vi "Configure Systems Copy.vi"() -> ()   [LabVIEW 2009, in "POLARIS BME DG.lvlib" / "BME_DG_System.lvclass"]
uses:
  DG Classes/BME_DG_System/BME_DG_System.lvclass
  DetectDG.ctl
  System DG Selection.ctl
  LV-BME Interface/BME_DG_TriggerSettings.ctl
  LV-BME Interface/ClockSource.ctl
  SG08_Settings.ctl
  LV-BME Interface/BME_DG_V2TriggerSettings.ctl
  MSBus.ctl
  LV-BME Interface/ChnlSettings.ctl
  Go_Done_Chnl_Settings.ctl
  SG08_Chnl_Settings.ctl
  Chnl Settings Complete.ctl
  Card Config.ctl
  <vilib>/Utility/xml.llb/Write to XML File(array).vi
  <vilib>/Utility/error.llb/DialogType.ctl
  POLARIS BME DG.lvlib
panel:
  in  "stop":bool
  in  "Tab Control":T1(tab)=enum."Define Channels"
  in  "InstalledDGs":T2[](array[typedef])
  in  "Select System":u16(ring) items=["MiraSync", "POLARISTrigger"]
  in  "Systems":T3[](array[typedef])
  in  "Selected DG":u16(ring) items=["0", "1", "2"]
  in  "Add":bool
  in  "Remove":bool
  in  "Empty Systems":bool
  in  "DetectDGs":bool
  in  "Find Card by Name":u16(ring) items=["MiraSync", "FE PP", "A1 Hapt", "A1 Neben", "A2 Haupt", "A2 Neben", "A2 PP", "A2 PP, A2.5", "A3 Haupt", "A4 Haupt"]
  in  "Card Config":T9(array[cluster]) {"Advanced Settings"."Trigger on MS Bus" format="%04x" items=["Local Primary0x1"=1, "Local Secondary0x2"=2, "Local Force 0x4"=4, "Resynchronize 0x8"=8, "Master Prim. 0x10"=16, "Master Sec. 0x20"=32, "Master Force  0x40"=64, "System Clock 0x80"=128, "Delay Clock 0x100"=256, "Inhibit Local 0x200"=512, "Start Local 0x400"=1024, "Start Bus 0x800"=2048, "Step Back Local 0x1000"=4096, "Step Back Bus 0x2000"=8192, "RunCircle 0x4000"=16384, "SyncReload 0x8000"=32768, "From E 0x10000"=65536, "From F 0x20000"=131072, "From Bus 0x40000"=262144]; "Advanced Settings"."Force Trigger (µs)" min=0.0 format="%.6f"; "SG08_Settings"."StepBackTime (µs)" min=0.0 format="%.6f"; "SG08_Settings"."Gate Delay (µs)" format="%.3f"; "SG08_Settings"."Gate Level" min=-2.5 max=2.5 format="%.3g"; "Base Settings"."Gate Divider" min=1 max=1000000; "Base Settings"."Clock Source" items=["Internal Oscillator"=1, "External Trigger"=2, "Trigger-> Oscillator"=3, "MasterSlave Bus"=4]; "Base Settings"."Inhibit(µs)" format="%#_11g"}
  in  "Find Card by Chnl":u16(ring) items=["MiraSyncT", "MiraSyncA", "MiraSyncB", "Delay Offset", "Pulspicker On", "Pulspicker Off", "10 Hz Target", "A1 PC On", "A1 PC Off", "Fast PC On", "Dazzler", "Kompressor", "A2 LDD", "A2 PC On", "A2 PC Off", "Oszi", "Kamera", "A5", "A2 PP1 On", "A2 PP1 Off", "A2 PP2 On", "A2 PP2 Off", "A2.5 LDD", "Keppis A3", "A3 LDD", "A3 PC On", "A3 PC Off", "A4 LDD", "A3-Kamera", "A4-Kamera", "Oszi", "A2 PP1 On", "A2 PP2 Off", "A3 LDD", "A4 LDD"]
  in  "Find Chnl":u16(ring) items=["MiraSyncT", "MiraSyncA", "MiraSyncB", "Delay Offset", "Pulspicker On", "Pulspicker Off", "10 Hz Target", "A1 PC On", "A1 PC Off", "Fast PC On", "Dazzler", "Kompressor", "A2 LDD", "A2 PC On", "A2 PC Off", "Oszi", "Kamera", "A5", "A2 PP1 On", "A2 PP1 Off", "A2 PP2 On", "A2 PP2 Off", "A2.5 LDD", "Keppis A3", "A3 LDD", "A3 PC On", "A3 PC Off", "A4 LDD", "A3-Kamera", "A4-Kamera", "Oszi", "A2 PP1 On", "A2 PP2 Off", "A3 LDD", "A4 LDD"]
  in  "Copy Chnl Names":bool=TRUE
  in  "Chnls":T13(array[cluster]) {"ChnParameter"."Delay (µs)" min=0.0 max=100000000.0 format="%.5f"; "G08_Chnl_Settings"."Pulse Width (µs)" min=0.0 max=8947840.0 format="%#.6f"; "Go and Done Signal"."Done Signal" format="%04x" items=["Local Primary"=1, "Local Secondary"=2, "Local Force"=4, "Master Primary"=16]; "Go and Done Signal"."Go Signal" format="%04x" items=["Local Primary0x1"=1, "Local Secondary0x2"=2, "Local Force 0x4"=4, "Resynchronize 0x8"=8, "Master Prim. 0x10"=16, "Master Sec. 0x20"=32, "Master Force  0x40"=64, "System Clock 0x80"=128, "Delay Clock 0x100"=256, "Inhibit Local 0x200"=512, "Start Local 0x400"=1024, "Start Bus 0x800"=2048, "Step Back Local 0x1000"=4096, "Step Back Bus 0x2000"=8192, "RunCircle 0x4000"=16384, "SyncReload 0x8000"=32768, "From E 0x10000"=65536, "From F 0x20000"=131072, "From Bus 0x40000"=262144]}
  out "Last Change":timestamp=timestamp(3422440183.453125 s since 1904-01-01)
  in  "Save":bool
  in  "Load":bool=TRUE
  in  "Config File":path
  # "DGNr"
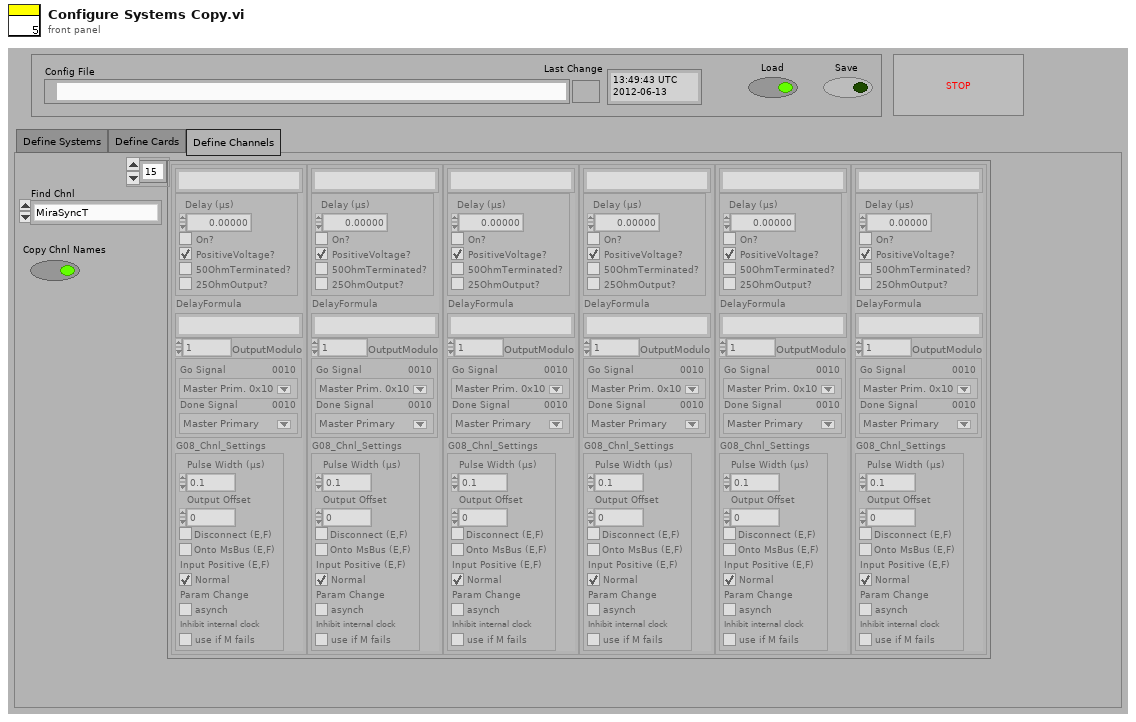
[diagram p1: front panel]
types:
  T1 = enum32{"Define Systems", "Define Cards", "Define Channels"}
  T2 = typedef "POLARIS BME DG.lvlib/DetectDG.ctl" = cluster{"DG_Number":i32, "DG_Product":i32, "Product Name":string, "Bus_Number":i32, "Slot_Number":i32, "Master":bool}
  T3 = typedef "POLARIS BME DG.lvlib/System DG Selection.ctl" = cluster{"Selected System DGs":T2[], "Name":string}
  T4 = typedef "POLARIS BME DG.lvlib/BME_DG_TriggerSettings.ctl" = cluster{"Clock Source":T5, " clock modulo":u32, "TriggerEnabled?":bool, "trigger modulo ":i32, "InputTerminated?":bool, "Inhibit(µs)":dbl, "TriggerLevel":dbl, "PresetValue":i32, "InternalTrigger?":bool, "InternalArm?":bool, "SWTrigger?":bool, "RisingEdge?":bool, "StopOnPreset?":bool, "ResetWhenDone?":bool, "Gate Divider":i32, "PositiveGate?":bool}
  T5 = typedef "POLARIS BME DG.lvlib/ClockSource.ctl" = i32
  T6 = typedef "POLARIS BME DG.lvlib/SG08_Settings.ctl" = cluster{"Gate Terminate":bool, "Gate Level":dbl, "Gate Delay (µs)":dbl, "StepBackTime (µs)":dbl, "Burst Counter":u32, "Trigger Divider":u32, "Trigger Multiplier":u32}
  T7 = typedef "POLARIS BME DG.lvlib/BME_DG_V2TriggerSettings.ctl" = cluster{"Trigger on MS Bus":T8, "Force Trigger (µs)":dbl, "Gate Type":bool, "Synchronize Gate":bool}
  T8 = typedef "POLARIS BME DG.lvlib/MSBus.ctl" = u32
  T9 = cluster{"Logical Name":string, "Base Settings":T4, "SG08_Settings":T6, "Channel Names":string[], "Advanced Settings":T7}[]
  T10 = typedef "POLARIS BME DG.lvlib/ChnlSettings.ctl" = cluster{" Delay (µs)":dbl, "On?":bool, "PositiveVoltage?":bool, "50OhmTerminated? ":bool, "25OhmOutput?":bool}
  T11 = typedef "POLARIS BME DG.lvlib/Go_Done_Chnl_Settings.ctl" = cluster{"Go Signal":T8, "Done Signal":u32}
  T12 = typedef "POLARIS BME DG.lvlib/SG08_Chnl_Settings.ctl" = cluster{"Pulse Width (µs)":dbl, "Output Offset":u32, "Disconnect (E,F)":bool, "Onto MsBus (E,F)":bool, "Input Positive (E,F)":bool, "Param Change":bool, "Inhibit internal clock":bool}
  T13 = cluster{"Channel Name":string, "ChnParameter":T10, "DelayFormula":string, "OutputModulo":i32, "Go and Done Signal":T11, "G08_Chnl_Settings":T12}[]
  T14 = typedef "POLARIS BME DG.lvlib/Chnl Settings Complete.ctl" = cluster{"Channel Name":string, "ChnParameter":T10, "DelayFormula":string, "OutputModulo":i32, "Go and Done Signal":T11, "G08_Chnl_Settings":T12}
  T15 = typedef "POLARIS BME DG.lvlib/Card Config.ctl" = cluster{"Logical Name":string, "Base Settings":T4, "SG08_Settings":T6, "Channel Names":string[], "Advanced Settings":T7}
  T16 = typedef "DialogType.ctl" = u16
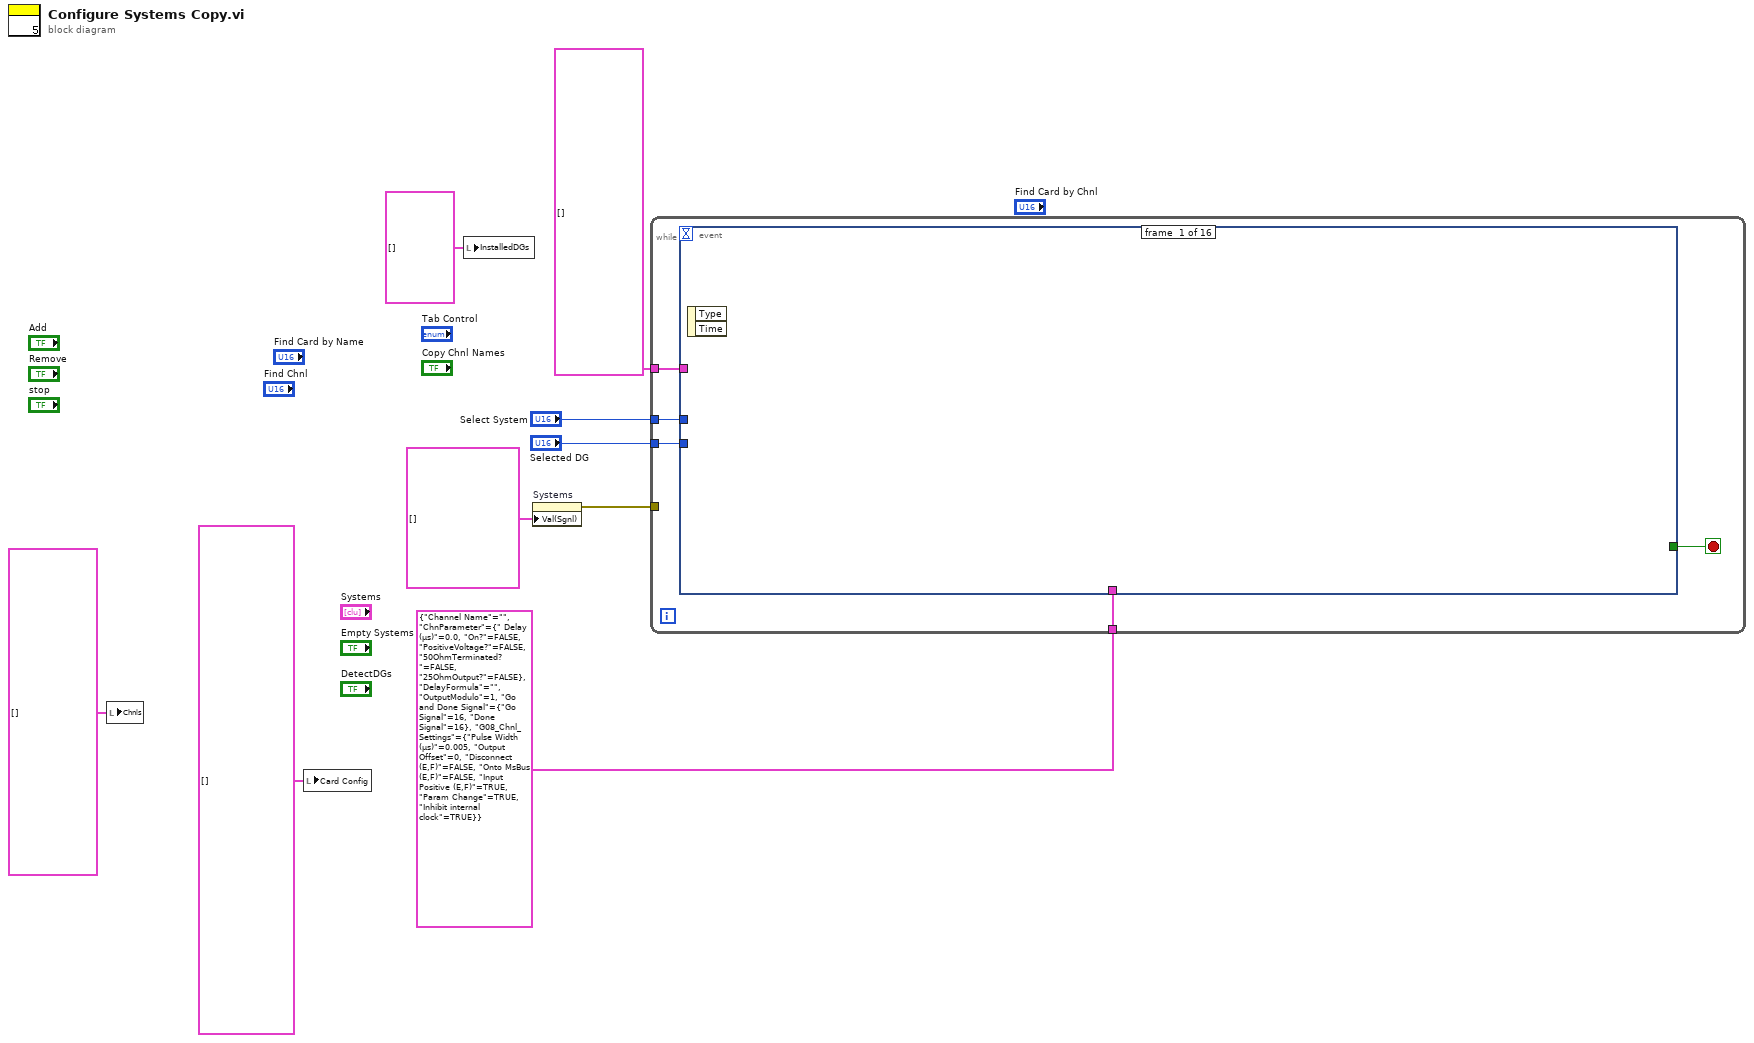
[diagram p0: block diagram]
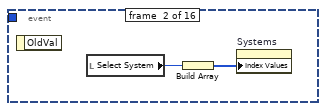
[diagram p2: hidden frame]
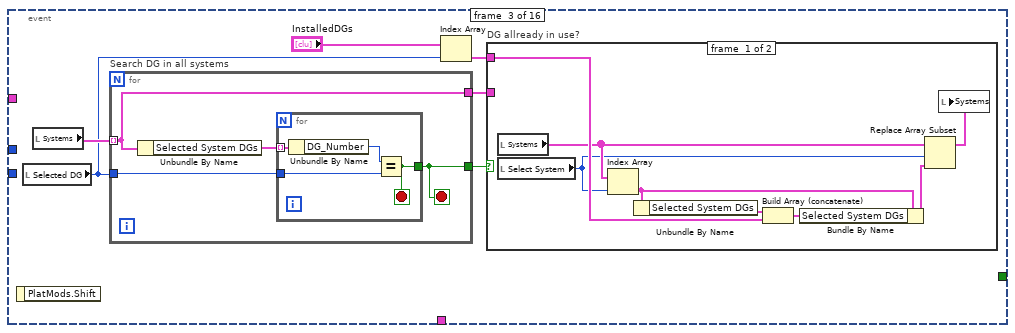
[diagram p3: hidden frame]
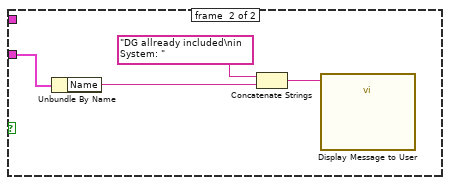
[diagram p4: hidden frame]
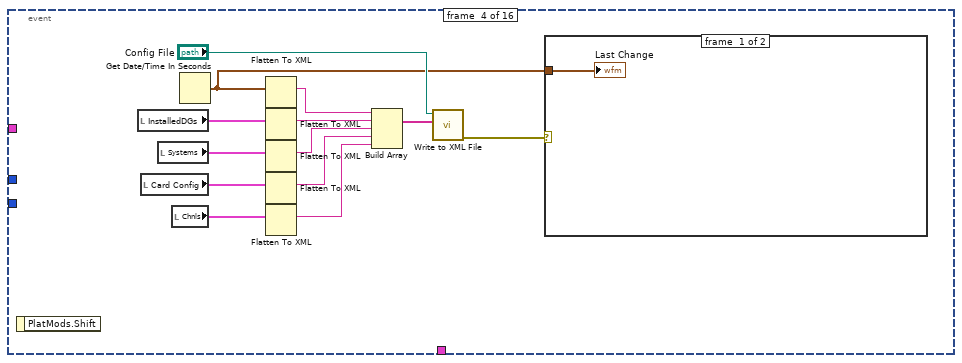
[diagram p5: hidden frame]
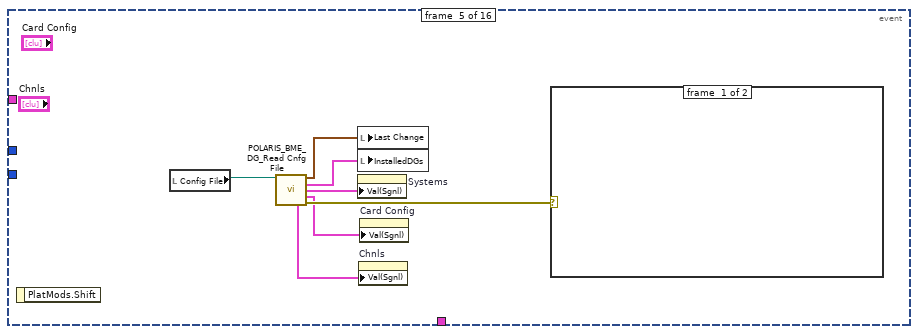
[diagram p7: hidden frame]
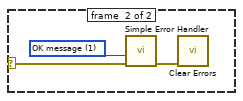
[diagram p8: hidden frame]
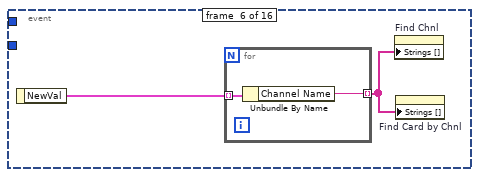
[diagram p9: hidden frame]
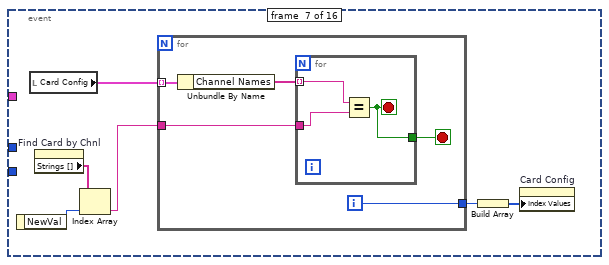
[diagram p10: hidden frame]
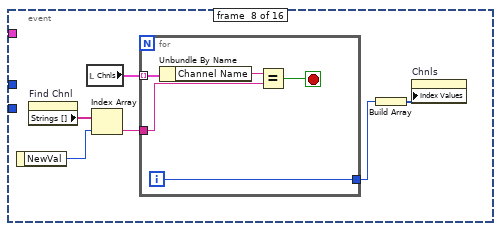
[diagram p11: hidden frame]
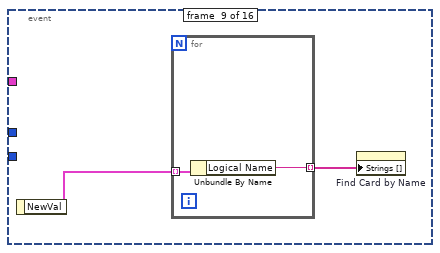
[diagram p12: hidden frame]
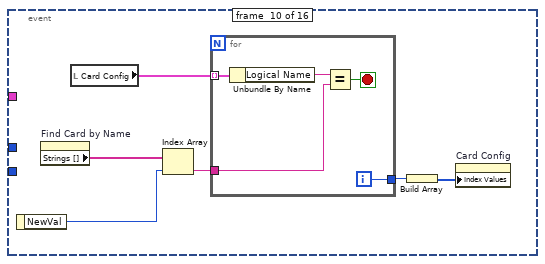
[diagram p13: hidden frame]
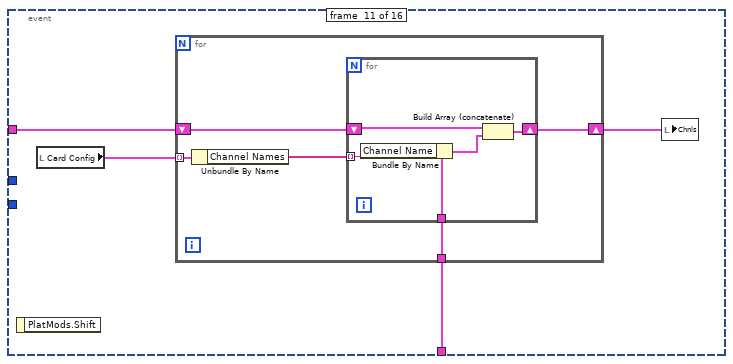
[diagram p14: hidden frame]
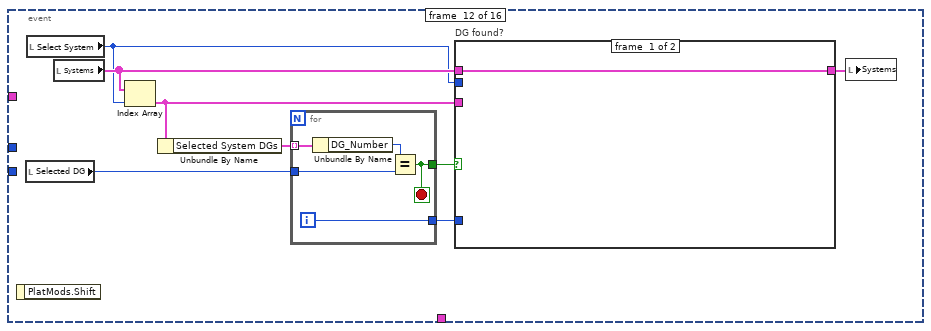
[diagram p15: hidden frame]
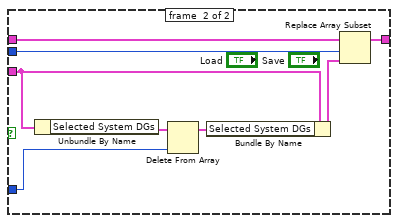
[diagram p16: hidden frame]
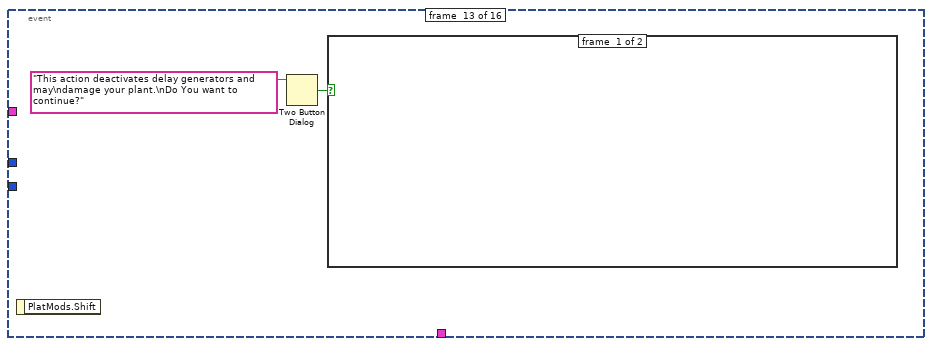
[diagram p17: hidden frame]
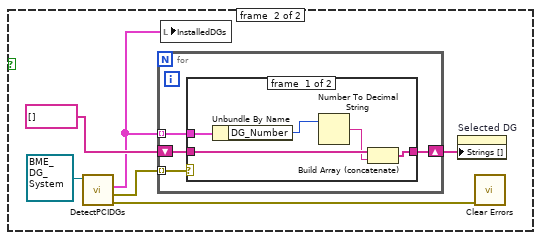
[diagram p18: hidden frame]
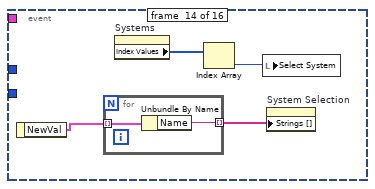
[diagram p20: hidden frame]
diagram:
  n1 = local write "Chnls"(T14[] [] ("Chnls")) -> ()
  n2 = local write "Card Config"(T15[] [] ("Card Config")) -> ()
  n3 = local write "InstalledDGs"(T2[] [] ("InstalledDGs")) -> ()
  n4 = property on="Systems" class="Arr (strict)"("Val(Sgnl)"=T3[] [] ("Value (Signaling)")) -> (error out=w6:errorcluster)  [unwired: 2 in, 1 out]
  n5 = while {
    tunnel: "Select System" -> [w13]
    tunnel: "Selected DG" -> [w12]
    tunnel: w6 -> [_]
    tunnel: T14 {"Channel Name"="", "ChnParameter"={" Delay (µs)"=0.0, "On?"=FALSE, "PositiveVoltage?"=FALSE, "50OhmTerminated? "=FALSE, "25OhmOutput?"=FALSE}, "DelayFormula"="", "OutputModulo"=1, "Go and Done Signal"={"Go Signal"=16, "Done Signal"=16}, "G08_Chnl_Settings"={"Pulse Width (µs)"=0.005, "Output Offset"=0, "Disconnect (E,F)"=FALSE, "Onto MsBus (E,F)"=FALSE, "Input Positive (E,F)"=TRUE, "Param Change"=TRUE, "Inhibit internal clock"=TRUE}} ("Cluster") -> [w11]
    tunnel: T14[] [] -> [w10]
    stop <- w14 stop-if-true
    n6 = event shown="[12] \"DetectDGs\": Mouse Down;  \"DetectDGs\": Key Down" {
      selector: _ -> [_ _ _ _ _ _ _ _ _ _ _ _ _ _ _ _]
      dyn-events: _ -> [_ _ _ _ _ _ _ _ _ _ _ _ _ _ _ _]
      timeout: _ -> [_ _ _ _ _ _ _ _ _ _ _ _ _ _ _ _]
      tunnel: [_ _ _ _ _ _ _ _ _ _ _ _ _ _ _ TRUE] -> w14
      tunnel: w13 -> [_ _ _ _ _ _ _ _ _ _ _ _ _ _ _ _]
      tunnel: w12 -> [_ _ _ _ _ _ _ _ _ _ _ _ _ _ _ _]
      tunnel: w11 -> [_ _ _ _ _ _ _ _ _ _ w112 _ _ _ _ _]
      tunnel: w10 -> [_ _ _ _ _ _ _ _ _ _ w111 _ _ _ _ _]
      event #0 {
        n7 = event-data() -> ()  [unwired: 1 in, 2 out]
      }
      event #1 {
        n8 = event-data() -> ()  [unwired: 1 in, 1 out]
        n9 = local read "Select System"() -> (w16:u16)
        n10 = Build Array(w16) -> (w15:u16[])
        n11 = property on="Systems" class="Arr (strict)"("Index Values"=w15) -> ()  [unwired: 2 in, 2 out]
      }
      event #2 {
        n12 = event-data() -> ()  [unwired: 1 in, 1 out]
        n13 = local read "Selected DG"() -> (w19:u16)
        n14 = local read "Systems"() -> (w22:T3[])
        n15 = for "Search DG in all systems" {
          tunnel: w22 -> [w35] mode=indexing
          tunnel: w19 -> [w37]
          tunnel: [w35] -> w20
          tunnel: [w36] -> w21
          stop <- w36 stop-if-true
          n16 = Unbundle By Name(w35) -> ("Selected System DGs"=w38:T2[])
          n17 = for {
            tunnel: w38 -> [w42] mode=indexing
            tunnel: w37 -> [w41]
            tunnel: [w39] -> w36
            stop <- w39 stop-if-true
            n18 = Unbundle By Name(w42) -> ("DG_Number"=w40:i32)
            n19 = Equal?(x=w40, y=w41) -> (x = y?=w39:bool)
          }
        }
        n20 = Index Array(array="InstalledDGs", index=w19) -> (element=w18:T2)
        n21 = case "DG allready in use?" shown="False" w21 {
          tunnel: w20 -> [_ w34]
          tunnel: w18 -> [w28 _]
          frame #0 {
            n22 = local read "Systems"() -> (w25:T3[])
            n23 = local read "Select System"() -> (w24:u16)
            n24 = Index Array(array=w25, index=w24) -> (element=w23:T3)
            n25 = Unbundle By Name(w23) -> ("Selected System DGs"=w30:T2[])
            n26 = Build Array (concatenate)(w30, w28) -> (w29:T2[])
            n27 = Bundle By Name(cluster=w23, "Selected System DGs"=w29) -> (w26:T3)
            n28 = Replace Array Subset(array=w25, new element=w26, index=w24) -> (w27:T3[])
            n29 = local write "Systems"(w27) -> ()
          }
          frame #1 {
            n30 = Unbundle By Name(w34) -> ("Name"=w31:string)
            n31 = Concatenate Strings("DG allready included\nin System: " ("string"), w31) -> (w33:string)
            n32 = call "Display Message to User"("Message"=w33) -> ()  [unwired: 9 in, 2 out]
          }
        }
      }
      event #3 {
        n33 = event-data() -> ()  [unwired: 1 in, 1 out]
        n34 = local read "InstalledDGs"() -> (w55:T2[])
        n35 = local read "Card Config"() -> (w46:T9)
        n36 = local read "Systems"() -> (w54:T3[])
        n37 = local read "Chnls"() -> (w44:T13)
        n38 = Get Date/Time In Seconds() -> (seconds since 1Jan1904=w48:timestamp)
        n39 = Flatten To XML(anything=w48) -> (xml string=w53:string)
        n40 = Flatten To XML(anything=w55) -> (xml string=w52:string)
        n41 = Flatten To XML(anything=w54) -> (xml string=w51:string)
        n42 = Flatten To XML(anything=w46) -> (xml string=w45:string)
        n43 = Flatten To XML(anything=w44) -> (xml string=w43:string)
        n44 = Build Array(w53, w52, w51, w45, w43) -> (w50:string[])
        n45 = call-poly <vilib>:"Write to XML File.vi"("XML Input"=w50, "XML File Path"="Config File") -> ("error out"=w47:errorcluster)  [unwired: 7 in, 2 out]
        n46 = case shown="No Error" w47 {
          tunnel: w48 -> [w56 _]
          frame #0 {
            "Last Change" <- w56
          }
          frame #1 {
          }
        }
      }
      event #4 {
        n47 = event-data() -> ()  [unwired: 1 in, 1 out]
        n48 = local read "Config File"() -> (w63:path)
        n49 = call "POLARIS_BME_DG_Read Cnfg File.vi"("Config File"=w63) -> ("Last Change"=w62:timestamp, "InstalledDGs"=w61:T2[], "DGSystems"=w60:T3[], "Cards"=w58:T15[], "Chnls"=w57:T14[], "error out"=w59:errorcluster)  [unwired: 9 in]
        n50 = local write "Last Change"(w62) -> ()
        n51 = local write "InstalledDGs"(w61) -> ()
        n52 = property on="Systems" class="Arr (strict)"("Val(Sgnl)"=w60) -> ()  [unwired: 2 in, 2 out]
        n53 = property on="Chnls" class="Arr (strict)"("Val(Sgnl)"=w57) -> ()  [unwired: 2 in, 2 out]
        n54 = property on="Card Config" class="Arr (strict)"("Val(Sgnl)"=w58) -> ()  [unwired: 2 in, 2 out]
        n55 = case shown="Error" w59 {
          selector: w59 -> [_ w66]
          frame #0 {
          }
          frame #1 {
            w64 = T16 1 items=["no dialog", "OK message", "continue or stop message", "OK message + warnings", "continue/stop + warnings"] ("type of dialog (OK msg:1)")
            n56 = call <vilib>:"Simple Error Handler.vi"("type of dialog (OK msg:1)"=w64, "error in (no error)"=w66) -> ("error out"=w65:errorcluster)  [unwired: 3 in, 4 out]
            n57 = call <vilib>:"Clear Errors.vi"("error in (no error)"=w65) -> ()  [unwired: 6 in, 1 out]
          }
        }
      }
      event #5 {
        n58 = event-data() -> ("NewVal"=w68:T13)  [unwired: 1 in]
        n59 = for {
          tunnel: w68 -> [w70] mode=indexing
          tunnel: [w69] -> w67 mode=indexing
          n60 = Unbundle By Name(w70) -> ("Channel Name"=w69:string)
        }
        n61 = property on="Find Chnl" class="Ring (strict)"("Strings []"=w67) -> ()  [unwired: 2 in, 2 out]
        n62 = property on="Find Card by Chnl" class="Ring (strict)"("Strings []"=w67) -> ()  [unwired: 2 in, 2 out]
      }
      event #6 {
        n63 = event-data() -> ("NewVal"=w75:u16)  [unwired: 1 in]
        n64 = local read "Card Config"() -> (w76:T9)
        n65 = property on="Find Card by Chnl" class="Ring (strict)"() -> ("Strings []"=w74:string[])  [unwired: 2 in, 2 out]
        n66 = Index Array(array=w74, index=w75) -> (element=w73:string)
        n67 = for {
          tunnel: w76 -> [w81] mode=indexing
          tunnel: w73 -> [w79]
          tunnel: [w78] -> w72
          i -> [w78]
          stop <- w77 stop-if-true
          n68 = Unbundle By Name(w81) -> ("Channel Names"=w80:string[])
          n69 = for {
            tunnel: w80 -> [w83] mode=indexing
            tunnel: w79 -> [w84]
            tunnel: [w82] -> w77
            stop <- w82 stop-if-true
            n70 = Equal?(x=w83, y=w84) -> (x = y?=w82:bool)
          }
        }
        n71 = Build Array(w72) -> (w71:i32[])
        n72 = property on="Card Config" class="Arr (strict)"("Index Values"=w71) -> ()  [unwired: 2 in, 2 out]
      }
      event #7 {
        n73 = event-data() -> ("NewVal"=w90:u16)  [unwired: 1 in]
        n74 = property on="Find Chnl" class="Ring (strict)"() -> ("Strings []"=w89:string[])  [unwired: 2 in, 2 out]
        n75 = local read "Chnls"() -> (w88:T13)
        n76 = Index Array(array=w89, index=w90) -> (element=w87:string)
        n77 = for {
          tunnel: w88 -> [w95] mode=indexing
          tunnel: w87 -> [w93]
          tunnel: [w91] -> w85
          i -> [w91]
          stop <- w92 stop-if-true
          n78 = Unbundle By Name(w95) -> ("Channel Name"=w94:string)
          n79 = Equal?(x=w94, y=w93) -> (x = y?=w92:bool)
        }
        n80 = Build Array(w85) -> (w86:i32[])
        n81 = property on="Chnls" class="Arr (strict)"("Index Values"=w86) -> ()  [unwired: 2 in, 2 out]
      }
      event #8 {
        n82 = event-data() -> ("NewVal"=w97:T9)  [unwired: 1 in]
        n83 = for {
          tunnel: w97 -> [w99] mode=indexing
          tunnel: [w98] -> w96 mode=indexing
          n84 = Unbundle By Name(w99) -> ("Logical Name"=w98:string)
        }
        n85 = property on="Find Card by Name" class="Ring (strict)"("Strings []"=w96) -> ()  [unwired: 2 in, 2 out]
      }
      event #9 {
        n86 = event-data() -> ("NewVal"=w101:u16)  [unwired: 1 in]
        n87 = property on="Find Card by Name" class="Ring (strict)"() -> ("Strings []"=w102:string[])  [unwired: 2 in, 2 out]
        n88 = local read "Card Config"() -> (w103:T9)
        n89 = Index Array(array=w102, index=w101) -> (element=w104:string)
        n90 = for {
          tunnel: w103 -> [w110] mode=indexing
          tunnel: w104 -> [w108]
          tunnel: [w106] -> w105
          i -> [w106]
          stop <- w107 stop-if-true
          n91 = Unbundle By Name(w110) -> ("Logical Name"=w109:string)
          n92 = Equal?(x=w109, y=w108) -> (x = y?=w107:bool)
        }
        n93 = Build Array(w105) -> (w100:i32[])
        n94 = property on="Card Config" class="Arr (strict)"("Index Values"=w100) -> ()  [unwired: 2 in, 2 out]
      }
      event #10 {
        n95 = event-data() -> ()  [unwired: 1 in, 1 out]
        n96 = local read "Card Config"() -> (w114:T9)
        n97 = for {
          tunnel: w114 -> [w119] mode=indexing
          shift-right: [w116] -> w113
          shift-left: w111 -> [w117]
          tunnel: w112 -> [w115]
          n98 = Unbundle By Name(w119) -> ("Channel Names"=w118:string[])
          n99 = for {
            tunnel: w118 -> [w121] mode=indexing
            shift-right: [w123] -> w116
            shift-left: w117 -> [w124]
            tunnel: w115 -> [w122]
            n100 = Bundle By Name(cluster=w122, "Channel Name"=w121) -> (w120:T14)
            n101 = Build Array (concatenate)(w124, w120) -> (w123:T14[])
          }
        }
        n102 = local write "Chnls"(w113) -> ()
      }
      event #11 {
        n103 = event-data() -> ()  [unwired: 1 in, 1 out]
        n104 = local read "Selected DG"() -> (w128:u16)
        n105 = local read "Select System"() -> (w125:u16)
        n106 = local read "Systems"() -> (w129:T3[])
        n107 = Index Array(array=w129, index=w125) -> (element=w126:T3)
        n108 = Unbundle By Name(w126) -> ("Selected System DGs"=w127:T2[])
        n109 = for {
          tunnel: w127 -> [w133] mode=indexing
          tunnel: w128 -> [w137]
          tunnel: [w136] -> w132
          tunnel: [w135] -> w131
          i -> [w135]
          stop <- w136 stop-if-true
          n110 = Unbundle By Name(w133) -> ("DG_Number"=w134:i32)
          n111 = Equal?(x=w134, y=w137) -> (x = y?=w136:bool)
        }
        n112 = case "DG found?" shown="True" w132 {
          tunnel: w131 -> [_ w143]
          tunnel: w129 -> [w138 w146]
          tunnel: [w138 w145] -> w130
          tunnel: w126 -> [_ w142]
          tunnel: w125 -> [_ w139]
          frame #0 {
          }
          frame #1 {
            n113 = Unbundle By Name(w142) -> ("Selected System DGs"=w144:T2[])
            n114 = Delete From Array(array=w144, index=w143) -> (array with subset deleted=w141:T2[])  [unwired: 1 in, 1 out]
            n115 = Bundle By Name(cluster=w142, "Selected System DGs"=w141) -> (w140:T3)
            n116 = Replace Array Subset(array=w146, new element=w140, index=w139) -> (w145:T3[])
          }
        }
        n117 = local write "Systems"(w130) -> ()
      }
      event #12 {
        n118 = event-data() -> ()  [unwired: 1 in, 1 out]
        n119 = Two Button Dialog(message="This action deactivates delay generators and may\ndamage your plant.\nDo You want to continue?") -> (T button?=w147:bool)  [unwired: 2 in]
        n120 = case shown="True" w147 {
          frame #0 {
          }
          frame #1 {
            n121 = call "DetectPCIDGs.vi"("BME_DG_System in"=refnum<class "BME_DG_System.lvclass"> refnum) -> ("error out"=w149:errorcluster, "Errors"=w152:errorcluster[], "InstalledDGs"=w150:T2[])  [unwired: 6 in, 2 out]
            n122 = for {
              tunnel: w152 -> [w155] mode=indexing
              tunnel: w150 -> [w157] mode=indexing
              shift-right: [w158] -> w153
              shift-left: string[] [] -> [w156]
              n123 = case shown="No Error" w155 {
                tunnel: [w163 w164] -> w158
                tunnel: w157 -> [w161 _]
                tunnel: w156 -> [w162 w164]
                frame #0 {
                  n124 = Unbundle By Name(w161) -> ("DG_Number"=w160:i32)
                  n125 = Number To Decimal String(number=w160) -> (decimal integer string=w159:string)  [unwired: 1 in]
                  n126 = Build Array (concatenate)(w162, w159) -> (w163:string[])
                }
                frame #1 {
                }
              }
            }
            n127 = local write "InstalledDGs"(w150) -> ()
            n128 = property on="Selected DG" class="Ring (strict)"("Strings []"=w153) -> ()  [unwired: 2 in, 2 out]
            n129 = call <vilib>:"Clear Errors.vi"("error in (no error)"=w149) -> ()  [unwired: 6 in, 1 out]
          }
        }
      }
      event #13 {
        n130 = event-data() -> ("NewVal"=w168:T3[])  [unwired: 1 in]
        n131 = for {
          tunnel: w168 -> [w170] mode=indexing
          tunnel: [w169] -> w167 mode=indexing
          n132 = Unbundle By Name(w170) -> ("Name"=w169:string)
        }
        n133 = property on="Systems" class="Arr (strict)"() -> ("Index Values"=w166:u32[])  [unwired: 2 in, 2 out]
        n134 = Index Array(array=w166) -> (element=w165:u32)  [unwired: 1 in]
        n135 = local write "Select System"(w165) -> ()
        n136 = property on="System Selection" class="Ring (strict)"("Strings []"=w167) -> ()  [unwired: 2 in, 2 out]
      }
      event #14 {
        n137 = event-data() -> ()  [unwired: 1 in, 1 out]
        n138 = Two Button Dialog(message="Are You sure???") -> (T button?=w171:bool)  [unwired: 2 in]
        n139 = case shown="True" w171 {
          frame #0 {
          }
          frame #1 {
            n140 = property on="Systems" class="Arr (strict)"("Val(Sgnl)"=T3[] [] ("Value (Signaling)")) -> ()  [unwired: 2 in, 2 out]
          }
        }
      }
      event #15 {
        n141 = event-data() -> ()  [unwired: 1 in, 1 out]
      }
    }
  }
